vi "Extract Source ID.vi"(4 "Payload in":string) -> (6 "Source ID":u32, 7 "Payload out":string)   [LabVIEW 2020, in "Vecto.lvlib" / "TCPMessaging.lvclass"]
uses:
  TCPMessaging.lvclass
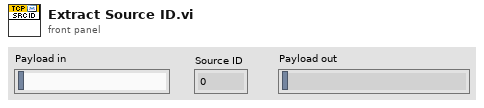
[diagram p1: front panel]
types:
  T1 = enum16{"big-endian, network order", "native, host order", "little-endian"}
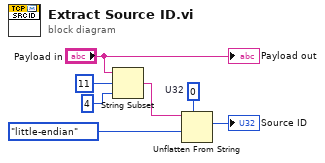
[diagram p0: block diagram]
diagram:
  w2 = u32 0  # U32
  n1 = String Subset(string="Payload in", offset (0)=11, length (rest)=4 ("length (rest)")) -> (substring=w4:string)
  n2 = Unflatten From String(type=w2, binary string=w4, byte order (0:big-endian, network order)=T1."little-endian") -> (value=→"Source ID":u32)  [unwired: 2 in, 2 out]
  "Payload out" <- "Payload in"
